vi "Profile_Max.vi"() -> (0 "New Values In":string[][](array[string])=[["Test data5"]], 1 "New Chs In":string[](array[string])=["30-10-03:New:Channel new5"])   [LabVIEW 2011]
uses:
  Results_plotter_Global.vi
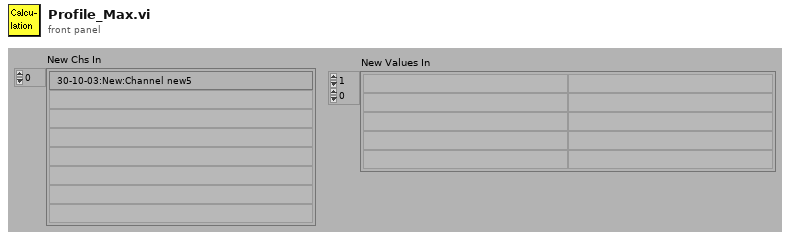
[diagram p1: front panel]
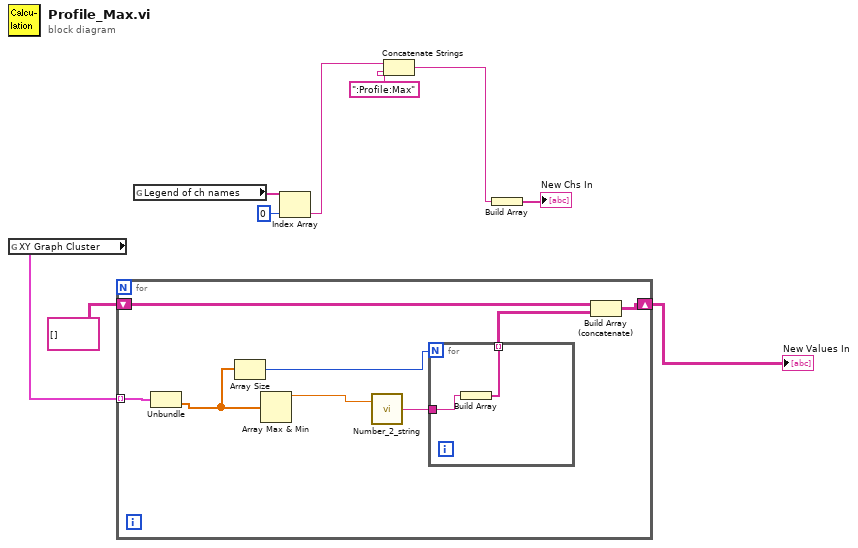
[diagram p0: block diagram]
diagram:
  n1 = global read "Results_plotter_Global.vi" "XY Graph Cluster"() -> (w8:cluster{dbl[], dbl[]}[])
  n2 = for {
    tunnel: w8 -> [w17] mode=indexing
    shift-right: [w15] -> w4
    shift-left: string[][] [] -> [w16]
    n3 = Unbundle(w17) -> (w13:dbl[])  [unwired: 1 out]
    n4 = Array Size(array=w13) -> (size(s)=w11:i32)
    n5 = Array Max & Min(array=w13) -> (max value=w14:dbl)  [unwired: 3 out]
    n6 = call "Number_2_string.vi"("number"=w14) -> ("String"=w12:string)  [unwired: 1 in]
    n7 = for {
      N: w11 -> [_]
      tunnel: w12 -> [w19]
      tunnel: [w18] -> w10 mode=indexing
      n8 = Build Array(w19) -> (w18:string[])
    }
    n9 = Build Array (concatenate)(w16, w10) -> (w15:string[][])
  }
  "New Values In" <- w4
  n10 = global read "Results_plotter_Global.vi" "Legend of ch names"() -> (w6:string[])
  n11 = Index Array(array=w6, index=0) -> (element=w2:string)
  n12 = Concatenate Strings(w2, ":Profile:Max" ("string")) -> (w1:string)
  n13 = Build Array(w1) -> (→"New Chs In":string[])
